vi "RT_userDIO_and_binning_time_to_FPGA.vi"(8 "error in (no error)":errorcluster) -> (0 "error out":errorcluster)   [LabVIEW 2020]
uses:
  PC_DIO_Cluster.ctl
  <vilib>/FPGAPlugInAG/cRIO-9040/niLvFpga_Open_cRIO-9040.vi
  <vilib>/Utility/error.llb/Error Cluster From Error Code.vi
  <vilib>/rvi/errors/niLvFpgaAdjustHostInterfaceError.vi
  <vilib>/rvi/interface/nirviOpenFPGA/nirviOpenFPGA.xnode
  FPGA Bitfiles/depapp_FPGATarget_FPGAmainsimplifi_zNZNOOeLYlY.lvbitx
  FPGA_main_simplified.vi
  <vilib>/rvi/interface/nirviReadWriteControl/nirviReadWriteControl.xnode
  NiFpgaLv.dll
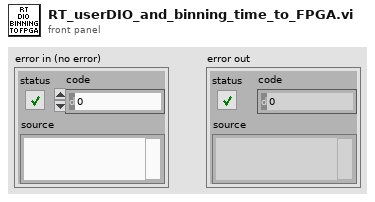
[diagram p1: front panel]
types:
  T1 = typedef "PC_DIO_Cluster.ctl" = cluster{"DIO1":bool, "DIO0":bool, "DIO2":bool, "DIO3":bool}
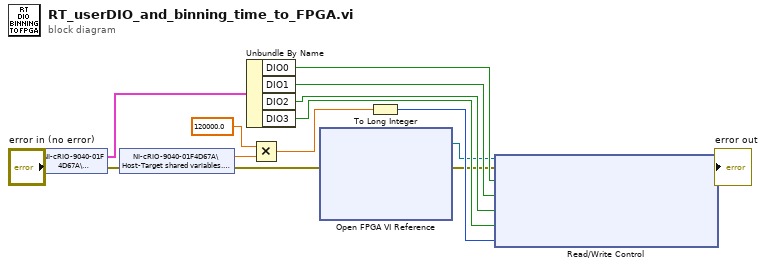
[diagram p0: block diagram]
diagram:
  n1 = shared-variable "NI-cRIO-9040-01F4D67A\\Host-Target shared variables.lvlib\\DIO"(error in="error in (no error)") -> (w1:T1, error out=w9:errorcluster)
  n2 = shared-variable "NI-cRIO-9040-01F4D67A\\Host-Target shared variables.lvlib\\Binning Time"(error in=w9) -> (w11:dbl, error out=w10:errorcluster)
  n3 = Unbundle By Name(w1) -> ("DIO0"=w5:bool, "DIO1"=w6:bool, "DIO2"=w7:bool, "DIO3"=w8:bool)
  n4 = Multiply(x=120000.0, y=w11) -> (x*y=w13:dbl)
  n5 = xnode "Open FPGA VI Reference"("error in"=w10) -> ("FPGA VI Reference Out"=w4:refnum<k20>, "error out"=w3:errorcluster)  [unwired: 1 in]
  n6 = To Long Integer(number=w13) -> (32bit integer=w14:i32)
  n7 = xnode "Read/Write Control"("FPGA VI Reference In"=w4, "error in"=w3, "DIO0"=w5, "DIO1"=w6, "DIO2"=w7, "DIO3"=w8, "Binning Time (ticks)"=w14) -> ("error out"=→"error out":errorcluster)  [unwired: 1 out]
